vi "camera control.vi"   [LabVIEW 2012, in "Sendmail.lvrbt"]
uses:
  Sendmail.lvrbt
  <vilib>/NXT/Block Support/NXT_MessageMailbox.ctl
  <vilib>/NXT/Hardware/Plugins/Tetrix 180 deg Servo/Tetrix180ServoAddress.ctl
  <vilib>/NXT/Dual Mode Library/BT/BlueTooth_Read_string.vi
  <vilib>/NXT/NXTIO Xnodes/NXTIONodeSubVIs/TETRIX IO Move Servos.vi
  <vilib>/NXT/Subs/LVHSConnector.ctl
  <vilib>/NXT/NXTIO Xnodes/AddressXNode/NXTIOAddress.xnode
  <vilib>/NXT/NXTIO Xnodes/NXTIOXNode/NXTIO.xnode
  <vilib>/NXT/LegoClasses/BrickReference/BrickReference.lvclass
types:
  T1 = typedef "Tetrix180ServoAddress.ctl" = i16
  T2 = cluster{"Tetrix180Servo":T1, "Tetrix180Servo 2":T1}
  T3 = typedef "NXT_MessageMailbox.ctl" = u8
  T4 = cluster{"Tetrix180Servo":T1, "Tetrix180Servo":T1}
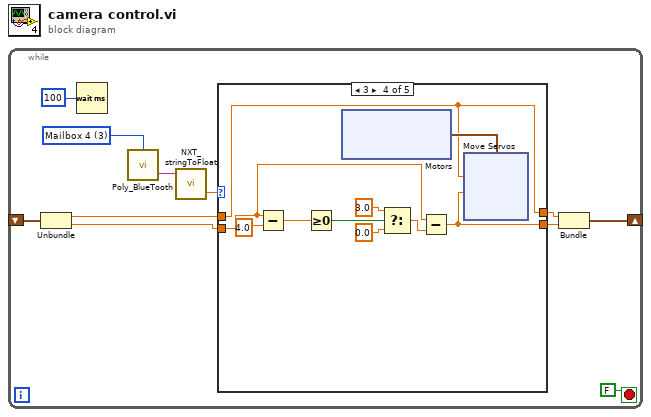
[diagram p0: block diagram]
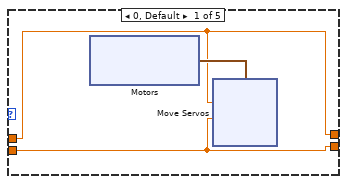
[diagram p2: hidden frame]
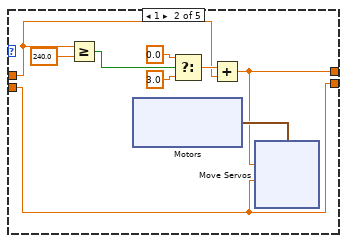
[diagram p3: hidden frame]
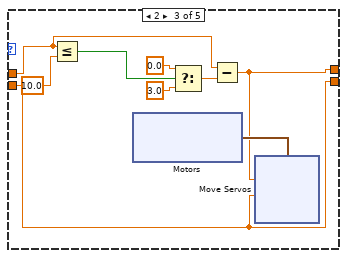
[diagram p4: hidden frame]
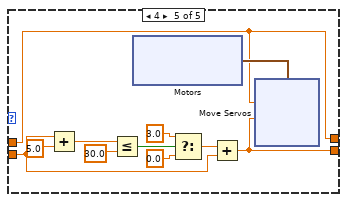
[diagram p5: hidden frame]
diagram:
  n1 = while {
    shift-right: [w6] -> _
    shift-left: _ -> [w5]
    stop <- FALSE stop-if-true
    w11 = T3 3 items=["Mailbox 1", "Mailbox 2", "Mailbox 3", "Mailbox 4", "Mailbox 5", "Mailbox 6", "Mailbox 7", "Mailbox 8", "Mailbox 9", "Mailbox 10"] ("Mailbox")
    n2 = Unbundle(w5) -> (w4:dbl, w3:dbl)
    n3 = Wait (ms)(milliseconds to wait=u32 100) -> ()  [unwired: 1 out]
    n4 = call-poly <vilib>:"Poly_BlueTooth.vi"("Mailbox"=w11) -> ("Message"=w10:string)  [unwired: 2 in, 1 out]
    n5 = call <vilib>:"NXT_stringToFloat.vi"("string"=w10) -> ("number"=w7:sgl)  [unwired: 2 in, 1 out]
    n6 = case shown="3" w7 {
      tunnel: w4 -> [w13 w26 w46 w68 w95]
      tunnel: w3 -> [w12 w33 w53 w66 w88]
      tunnel: [w13 w29 w49 w68 w95] -> w2
      tunnel: [w12 w33 w53 w69 w87] -> w1
      frame 0, Default {
        n7 = xnode "Motors"() -> ("Motor"=w14:T4)
        n8 = xnode "Move Servos"("Position 2"=w12, "Position 1"=w13, "Servos"=w14) -> ()  [unwired: 1 in, 1 out]
      }
      frame 1 {
        n9 = Greater Or Equal?(x=w26, y=240.0) -> (x >= y?=w27:bool)
        n10 = xnode "Motors"() -> ("Motor"=w34:T4)
        n11 = Select(t=0.0, s=w27, f=3.0) -> (s? t:f=w30:dbl)
        n12 = Add(x=w30, y=w26) -> (x+y=w29:dbl)
        n13 = xnode "Move Servos"("Position 2"=w33, "Position 1"=w29, "Servos"=w34) -> ()  [unwired: 1 in, 1 out]
      }
      frame 2 {
        n14 = Less Or Equal?(x=w46, y=10.0) -> (x <= y?=w47:bool)
        n15 = xnode "Motors"() -> ("Motor"=w54:T4)
        n16 = Select(t=0.0, s=w47, f=3.0) -> (s? t:f=w50:dbl)
        n17 = Subtract(x=w46, y=w50) -> (x-y=w49:dbl)
        n18 = xnode "Move Servos"("Position 2"=w53, "Position 1"=w49, "Servos"=w54) -> ()  [unwired: 1 in, 1 out]
      }
      frame 3 {
        n19 = Subtract(x=w66, y=4.0) -> (x-y=w73:dbl)
        n20 = Greater Or Equal To 0?(x=w73) -> (x >= 0?=w72:bool)
        n21 = xnode "Motors"() -> ("Motor"=w75:T4)
        n22 = Select(t=3.0, s=w72, f=0.0) -> (s? t:f=w67:dbl)
        n23 = Subtract(x=w66, y=w67) -> (x-y=w69:dbl)
        n24 = xnode "Move Servos"("Position 2"=w69, "Position 1"=w68, "Servos"=w75) -> ()  [unwired: 1 in, 1 out]
      }
      frame 4 {
        n25 = Add(x=w88, y=5.0) -> (x+y=w94:dbl)
        n26 = Less Or Equal?(x=w94, y=30.0) -> (x <= y?=w92:bool)
        n27 = xnode "Motors"() -> ("Motor"=w97:T4)
        n28 = Select(t=3.0, s=w92, f=0.0) -> (s? t:f=w89:dbl)
        n29 = Add(x=w89, y=w88) -> (x+y=w87:dbl)
        n30 = xnode "Move Servos"("Position 2"=w87, "Position 1"=w95, "Servos"=w97) -> ()  [unwired: 1 in, 1 out]
      }
    }
    n31 = Bundle(w2, w1) -> (w6:cluster{dbl, dbl})  [unwired: 1 in]
  }
